vi "AprilTag Target Package.vi"() -> ()   [LabVIEW 2023]
uses:
  Camera Info.ctl
  AprialTag Main Cluster.ctl
  AprialTag States.ctl
  <vilib>/vision/Image Controls.llb/IMAQ Image.ctl
  Camera Set Up/Event Setup Types.ctl
  <vilib>/Utility/config.llb/Read Key (String).vi
  <vilib>/Utility/config.llb/Write Key (String).vi
  <vilib>/Utility/config.llb/NI_LVConfig.lvlib
panel:
  in  "Main":enum32{"Page 1", "Page 2"}(tab)
  out "Tag ID":dbl[](array[numeric]) caption="Tag Number"
  out "Image":T1(plugin-control)
  in  "Camera Name":string="cam0"
  in  "Settings":bool
  in  "Save":bool
  in  "Tools":bool
  out "Fps":dbl format="%#.0f"
  out "Distance":dbl[](array[numeric]) format="%.1f"
  out "Angle":dbl[](array[numeric]) format="%.1f"
  in  "Home":bool
  in  "FOV":dbl=68.5
  in  "Robot Calibration Cluster":T2={"Camera Height on robot (in)"=9.5, "Camera Angle on the robot (deg)"=2.5, "Camera FOV Top to Bottom View Angle (deg)"=26.5, "Target size (in)"=6.5, "Distance to front of bumper (in)"=9.75} {"Distance to front of bumper (in)" format="%#_13g"; "Target size (in)" format="%#_13g"; "Camera FOV Top to Bottom View Angle (deg)" format="%#_13g"; "Camera Angle on the robot (deg)" format="%#_13g"; "Camera Height on robot (in)" format="%#_13g"}
  # "Edit the camera name to the camera that you are going to use for this target package"
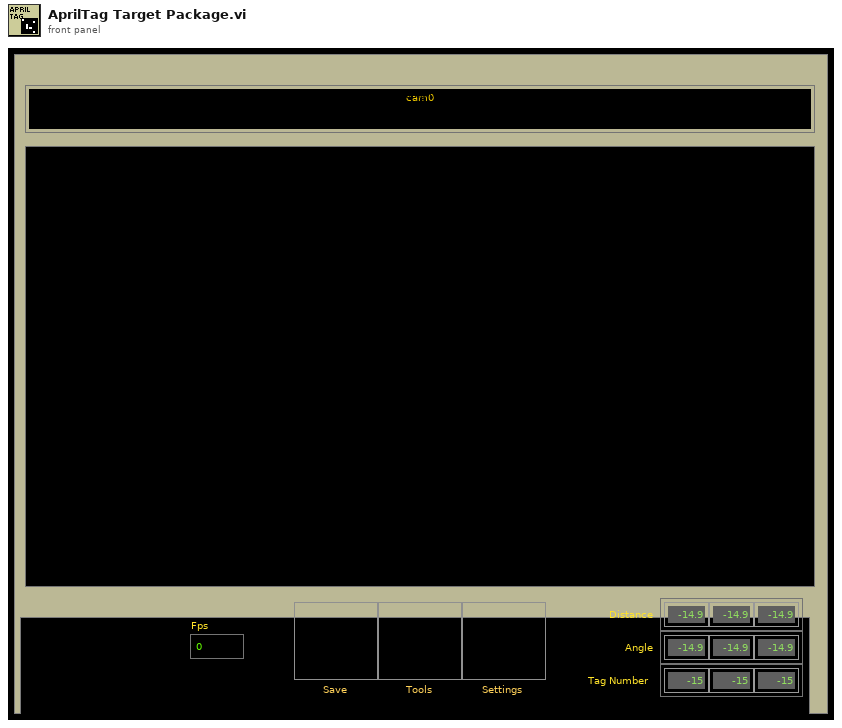
[diagram p1: front panel]
types:
  T1 = typedef "IMAQ Image.ctl" = refnum<image>
  T2 = typedef "Camera Info.ctl" = cluster{"Camera Height on robot (in)":dbl, "Camera Angle on the robot (deg)":dbl, "Camera FOV Top to Bottom View Angle (deg)":dbl, "Target size (in)":dbl, "Distance to front of bumper (in)":dbl}
  T3 = typedef "AprialTag States.ctl" = enum16{"Message Dispatcher", "INI", "Open", "Save", "Exit"}
  T4 = typedef "AprialTag Main Cluster.ctl" = cluster{"AprilTage FIFO":T3[], "Camera Name":string, "AprilTag path":path, "Control Ref's":refnum<vi>[], "Greyscale Mask Image":T1, "Main Image":T1}
  T5 = typedef "Event Setup Types.ctl" = enum16{"Default", "Camera Loop Started", "Save Data", "Open Front Panel", "Exit"}
  T6 = typedef "Image Type" = u32
  T7 = cluster{"tag ID":i32, "Center":cluster{"X":dbl, "Y":dbl}, "homography matrix":dbl[], "decision margin":dbl, "Hamming Dist":i32, "corner points":cluster{"X":dbl, "Y":dbl}[], "Tag Family":string}[]
  T8 = typedef "AprilTag Target Fields.ctl" = cluster{"diameter points":cluster{"first point":cluster{"x":dbl, "y":dbl}, "projected point":cluster{"x":dbl, "y":dbl}}, "normalized center":cluster{"x":dbl, "y":dbl}, "Overall Score":dbl, "Distance (ft)":dbl, "Target corner points":cluster{"X":dbl, "Y":dbl}[], "Target Center":cluster{"X":dbl, "Y":dbl}}
  T9 = typedef "NI_LVConfig.lvlib/Config Data RefNum.ctl" = refnum<k1>
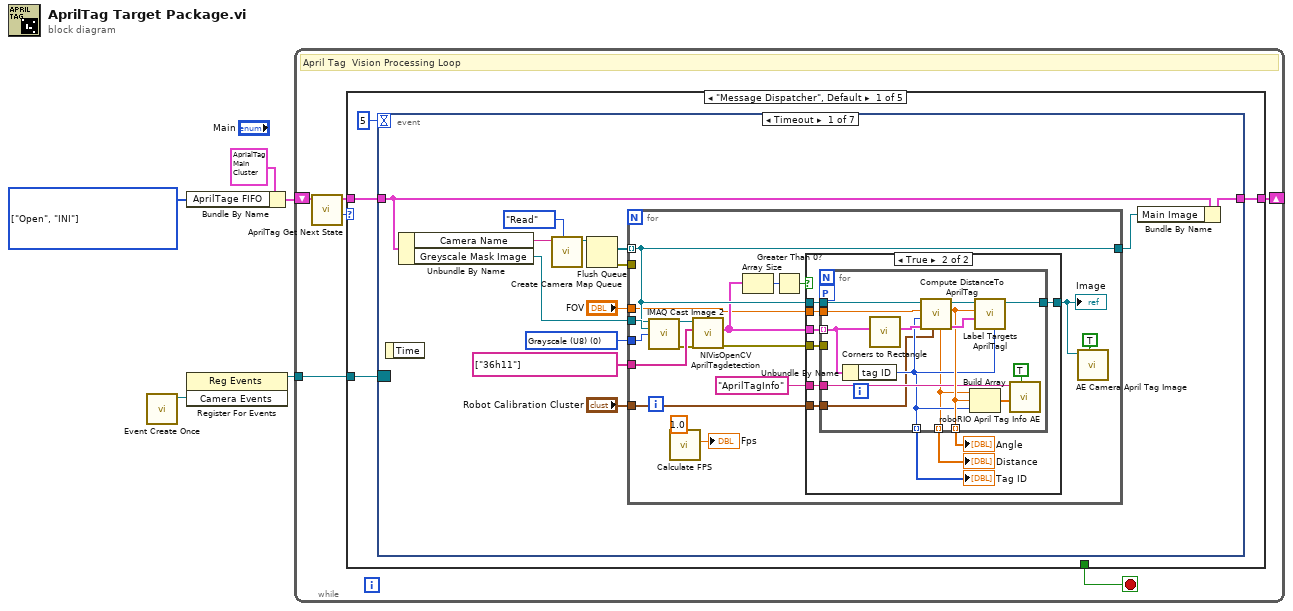
[diagram p0: block diagram]
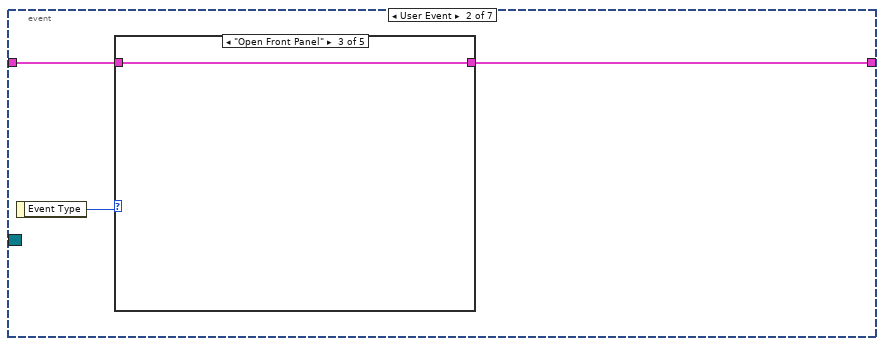
[diagram p3: hidden frame]
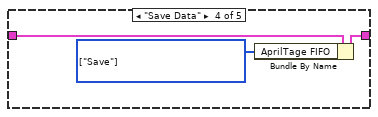
[diagram p6: hidden frame]
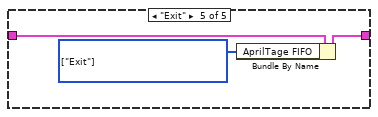
[diagram p7: hidden frame]
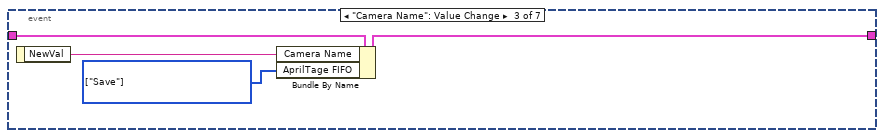
[diagram p8: hidden frame]
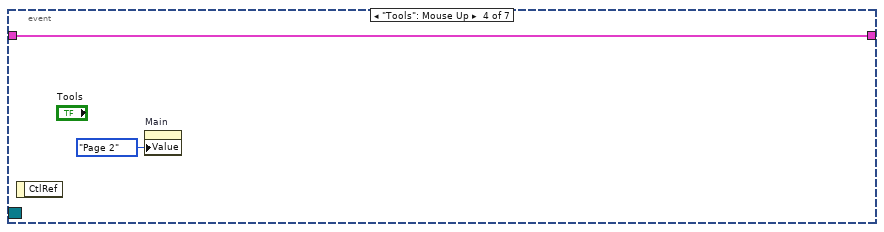
[diagram p9: hidden frame]
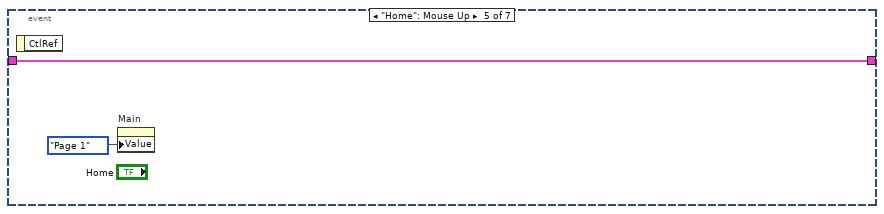
[diagram p10: hidden frame]
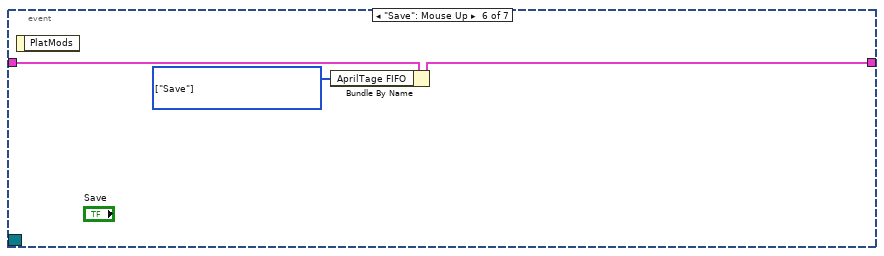
[diagram p11: hidden frame]
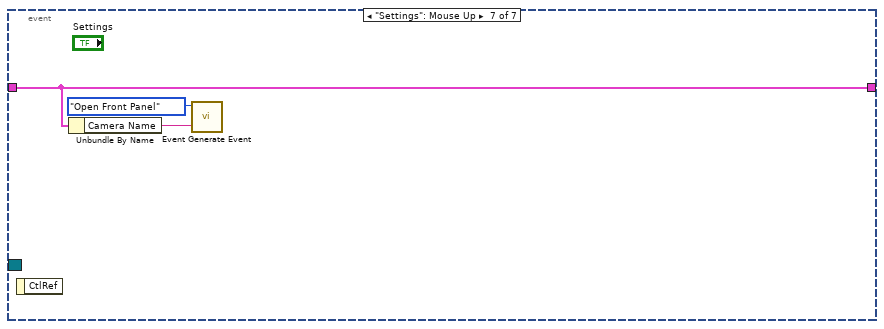
[diagram p12: hidden frame]
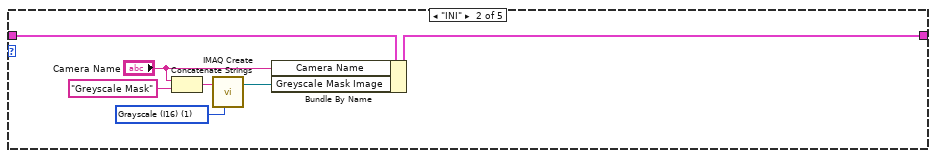
[diagram p13: hidden frame]
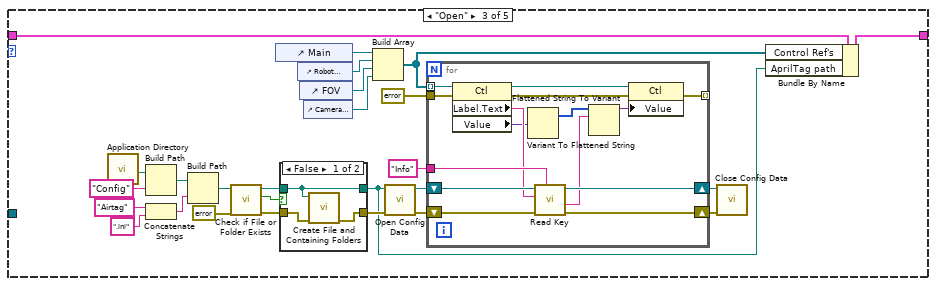
[diagram p14: hidden frame]
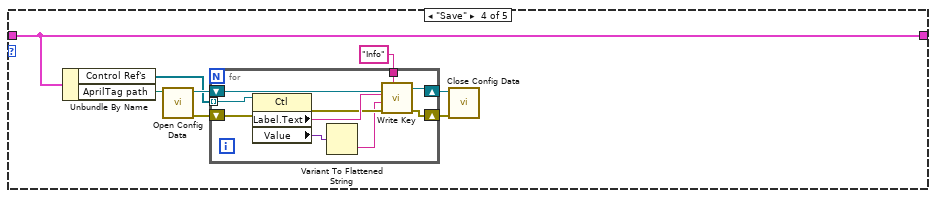
[diagram p16: hidden frame]
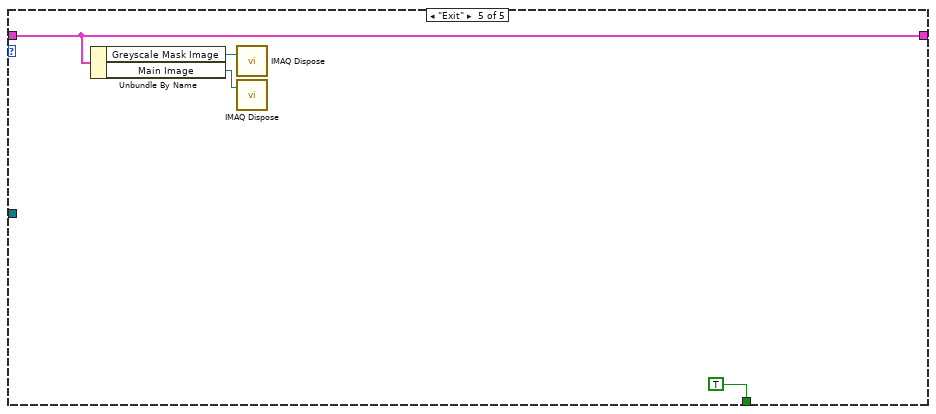
[diagram p17: hidden frame]
diagram:
  w1 = T3[] [enum."Open", enum."INI"] items=["Message Dispatcher", "INI", "Open", "Save", "Exit"] ("AprilTage FIFO")
  n1 = call "Event Create Once.vi"() -> ("Camera Events"=w5:refnum<user-event>)  [unwired: 10 in, 1 out]
  n2 = Bundle By Name(cluster=T4 {"AprilTage FIFO"=[], "Camera Name"="", "AprilTag path"=path "", "Control Ref's"=[], "Greyscale Mask Image"=refnum, "Main Image"=refnum} ("AprilTag Main Cluster out"), "AprilTage FIFO"=w1) -> (w2:T4)
  n3 = register-events(w5) -> (reference out=w4:refnum<event-registration>)  [unwired: 2 in, 1 out]
  n4 = while {
    tunnel: w4 -> [w11]
    shift-right: [w6] -> _
    shift-left: w2 -> [w9]
    stop <- w10 stop-if-true
    # "April Tag  Vision Processing Loop"
    n5 = call "AprilTag Get Next State.vi"("AprilTag Main Cluster in"=w9) -> ("Next State"=w7:T3, "AprilTag Main Cluster out"=w8:T4)  [unwired: 9 in]
    n6 = case shown="\"Message Dispatcher\", Default" w7 {
      tunnel: w11 -> [w15 _ _ _ _]
      tunnel: [_ _ _ _ TRUE] -> w10
      tunnel: w8 -> [w13 w103 w115 w153 w170]
      tunnel: [w12 w102 w113 w153 w170] -> w6
      frame "Message Dispatcher", Default {
        n7 = event shown="[0] Timeout" {
          selector: w15 -> [_ _ _ _ _ _ _]
          dyn-events: _ -> [_ _ _ _ _ _ _]
          timeout: 5 -> [_ _ _ _ _ _ _]
          tunnel: w13 -> [w21 w73 w86 w87 w89 w93 w95]
          tunnel: [w18 w72 w85 w87 w89 w92 w95] -> w12
          event Timeout {
            w26 = T6 0 items=["Grayscale (U8)", "Grayscale (I16)", "Grayscale (SGL)", "Complex (CSG)", "RGB (U32)", "HSL (U32)", "RGB (U64)", "Grayscale (U16)"] ("Image Type")
            n8 = event-data() -> ()  [unwired: 1 in, 1 out]
            n9 = Unbundle By Name(w21) -> ("Camera Name"=w20:string, "Greyscale Mask Image"=w19:T1)
            n10 = call "Create Camera Map Queue.vi"("Action"=enum16{"Read", "Write"}."Read", "Camera"=w20) -> ("value"=w27:refnum<queue>)  [unwired: 8 in, 1 out]
            n11 = Flush Queue(queue=w27) -> (remaining elements=w25:T1[], error out=w16:errorcluster)  [unwired: 1 in, 1 out]
            n12 = for {
              tunnel: w19 -> [w45]
              tunnel: w25 -> [w43] mode=indexing
              tunnel: w26 -> [w44]
              tunnel: [w43] -> w17
              tunnel: string[] ["36h11"] ("Tag Familys") -> [w42]
              tunnel: "FOV" -> [w33]
              tunnel: "Robot Calibration Cluster" -> [w32]
              tunnel: w16 -> [_]
              n13 = call "IMAQ Cast Image 2"("Image Src"=w43, "Image Dst"=w45, "Image Type"=w44) -> ("Image Dst Out"=w41:T1, "error out"=w36:errorcluster)  [unwired: 11 in]
              n14 = call "Calculate FPS.vi"("Frames Processed"=1.0) -> ("Fps"=→"Fps":dbl)  [unwired: 10 in]
              n15 = call "NIVisOpenCV AprilTagdetection.vi"("error in (no error)"=w36, "Tag Familys"=w42, "Image Src"=w41) -> ("error out"=w35:errorcluster, "Detected Tags"=w39:T7)  [unwired: 5 in, 2 out]
              n16 = Array Size(array=w39) -> (size(s)=w38:i32)
              n17 = Greater Than 0?(x=w38) -> (x > 0?=w37:bool)
              n18 = case shown="True" w37 {
                tunnel: w43 -> [w46 w56]
                tunnel: w39 -> [_ w55]
                tunnel: [w46 w54] -> w40
                tunnel: w35 -> [_ w53]
                tunnel: "AprilTagInfo" ("Name") -> [_ w49]
                tunnel: w33 -> [_ w48]
                tunnel: w32 -> [_ w47]
                frame False {
                }
                frame True {
                  n19 = for {
                    tunnel: w55 -> [w68] mode=indexing
                    tunnel: w56 -> [w69]
                    tunnel: [w70] -> w54
                    tunnel: w53 -> [_]
                    tunnel: [w59] -> w52 mode=indexing
                    tunnel: [w57] -> w51 mode=indexing
                    tunnel: [w63] -> w50 mode=indexing
                    tunnel: w49 -> [w61]
                    tunnel: w48 -> [w60]
                    tunnel: w47 -> [w58]
                    workers-P: _ -> [_]
                    n20 = Unbundle By Name(w68) -> ("tag ID"=w59:i32)
                    n21 = call "Corners to Rectangle.vi"("tag info"=w68) -> ("output cluster"=w67:T8)  [unwired: 10 in]
                    n22 = call "Compute DistanceTo AprilTag.vi"("Robot Calibration Cluster"=w58, "results"=w67, "AprilTag Number"=w59, "FOV Left to Right (deg)"=w60, "Image Src"=w69) -> ("results out"=w66:T8, "Offset Angle"=w63:dbl, "Image Dst Out"=w65:T1, "Distance from target (in)"=w57:dbl)  [unwired: 3 in]
                    n23 = Build Array(w57, w63, w59) -> (w62:dbl[])
                    n24 = call "Label Targets AprilTagl.vi"("AprilTag Number"=w59, "results"=w66, "Angle"=w63, "Image in"=w65) -> ("Image out"=w70:T1)  [unwired: 7 in]
                    n25 = call "roboRIO April Tag Info AE.vi"("Update"=TRUE, "Info in"=w62, "name"=w61) -> ()  [unwired: 8 in, 1 out]
                  }
                  "Distance" <- w51
                  "Angle" <- w50
                  "Tag ID" <- w52
                }
              }
              "Image" <- w40
              n26 = call "AE Camera April Tag Image.vi"("Update"=TRUE, "Ball Image in"=w40) -> ()  [unwired: 9 in, 1 out]
            }
            n27 = Bundle By Name(cluster=w21, "Main Image"=w17) -> (w18:T4)
          }
          event User Event {
            n28 = event-data() -> ("Event Type"=w71:T5)  [unwired: 1 in]
            n29 = case shown="\"Open Front Panel\"" w71 {
              tunnel: w73 -> [w74 w75 w76 w79 w82]
              tunnel: [w74 w75 w76 w78 w81] -> w72
              frame "Default" {
              }
              frame "Camera Loop Started" {
              }
              frame "Open Front Panel" {
              }
              frame "Save Data" {
                w77 = T3[] [enum."Save"] items=["Message Dispatcher", "INI", "Open", "Save", "Exit"] ("AprilTage FIFO")
                n30 = Bundle By Name(cluster=w79, "AprilTage FIFO"=w77) -> (w78:T4)
              }
              frame "Exit" {
                w80 = T3[] [enum."Exit"] items=["Message Dispatcher", "INI", "Open", "Save", "Exit"] ("AprilTage FIFO")
                n31 = Bundle By Name(cluster=w82, "AprilTage FIFO"=w80) -> (w81:T4)
              }
            }
          }
          event "Camera Name": Value Change {
            w84 = T3[] [enum."Save"] items=["Message Dispatcher", "INI", "Open", "Save", "Exit"] ("AprilTage FIFO")
            n32 = event-data() -> ("NewVal"=w83:string)  [unwired: 1 in]
            n33 = Bundle By Name(cluster=w86, "Camera Name"=w83, "AprilTage FIFO"=w84) -> (w85:T4)
          }
          event "Tools": Mouse Up {
            n34 = event-data() -> ()  [unwired: 1 in, 1 out]
            n35 = property on="Main" class="TabCtl (strict)"("Value"=enum32{"Page 1", "Page 2"}."Page 2" ("Main")) -> ()  [unwired: 2 in, 2 out]
          }
          event "Home": Mouse Up {
            n36 = event-data() -> ()  [unwired: 1 in, 1 out]
            n37 = property on="Main" class="TabCtl (strict)"("Value"=enum32{"Page 1", "Page 2"}."Page 1" ("Main")) -> ()  [unwired: 2 in, 2 out]
          }
          event "Save": Mouse Up {
            w91 = T3[] [enum."Save"] items=["Message Dispatcher", "INI", "Open", "Save", "Exit"] ("AprilTage FIFO")
            n38 = event-data() -> ()  [unwired: 1 in, 1 out]
            n39 = Bundle By Name(cluster=w93, "AprilTage FIFO"=w91) -> (w92:T4)
          }
          event "Settings": Mouse Up {
            n40 = event-data() -> ()  [unwired: 1 in, 1 out]
            n41 = Unbundle By Name(w95) -> ("Camera Name"=w94:string)
            n42 = call "Event Generate Event.vi"("Camera Name"=w94, "Event Type"=Event_Setup_Types."Open Front Panel") -> ()  [unwired: 10 in]
          }
        }
      }
      frame "INI" {
        w99 = T6 1 items=["Grayscale (U8)", "Grayscale (I16)", "Grayscale (SGL)", "Complex (CSG)", "RGB (U32)", "HSL (U32)", "RGB (U64)", "Grayscale (U16)"] ("Image Type")
        n43 = Concatenate Strings("Camera Name", "Greyscale Mask" ("string")) -> (w100:string)
        n44 = call "IMAQ Create"("Image Name"=w100, "Image Type"=w99) -> ("New Image"=w98:T1)  [unwired: 2 in, 2 out]
        n45 = Bundle By Name(cluster=w103, "Camera Name"="Camera Name", "Greyscale Mask Image"=w98) -> (w102:T4)
      }
      frame "Open" {
        n46 = call <vilib>:"Application Directory.vi"() -> ("Application Directory"=w118:path)
        n47 = Build Path(base path=w118, name or relative path="Config") -> (appended path=w116:path)
        n48 = Concatenate Strings("Airtag" ("string"), ".ini" ("name or relative path")) -> (w129:string)
        n49 = Build Path(base path=w116, name or relative path=w129) -> (appended path=w109:path)
        n50 = call <vilib>:"Check if File or Folder Exists.vi"("error in (no error)"=errorcluster {"status"=FALSE, "code"=0, "source"=""}, "path"=w109) -> ("error out"=w105:errorcluster, "file or folder exists?"=w107:bool, "dup path"=w108:path)  [unwired: 7 in]
        n51 = control-ref of="Main"() -> (w124:refnum<vi>)
        n52 = case shown="False" w107 {
          tunnel: [w132 w133] -> w119
          tunnel: w108 -> [w131 w134]
          tunnel: [w131 w134] -> w106
          tunnel: w105 -> [w130 w133]
          frame False {
            n53 = call <vilib>:"Create File and Containing Folders.vi"("error in (no error)"=w130, "file path"=w131) -> ("error out"=w132:errorcluster)  [unwired: 8 in, 1 out]
          }
          frame True {
          }
        }
        n54 = control-ref of="Robot Calibration Cluster"() -> (w123:refnum<vi>)
        n55 = control-ref of="FOV"() -> (w122:refnum<vi>)
        n56 = control-ref of="Camera Name"() -> (w114:refnum<vi>)
        n57 = Build Array(w124, w123, w122, w114) -> (w112:refnum<vi>[])
        n58 = call <vilib>:"Open Config Data.vi"("error in (no error)"=w119, "configuration file path"=w106) -> ("error out"=w125:errorcluster, "refnum"=w128:T9)  [unwired: 7 in, 1 out]
        n59 = for {
          tunnel: "Info" ("Camera Name") -> [w146]
          tunnel: w112 -> [w144] mode=indexing
          shift-right: [w148] -> w127
          shift-left: w128 -> [w149]
          shift-right: [w147] -> w126
          shift-left: w125 -> [w145]
          tunnel: [w139] -> _ mode=indexing
          tunnel: errorcluster {"status"=FALSE, "code"=0, "source"=""} ("error out") -> [w138]
          n60 = property class="Ctl"(reference=w144, error in=w138) -> (reference out=w142:refnum<vi>, error out=w140:errorcluster, "Label.Text"=w143:string, "Value"=w136:variant)
          n61 = Variant To Flattened String(Variant=w136) -> (1:w135:i16[])  [unwired: 1 out]
          n62 = call-poly <vilib>:"Read Key.vi"("section"=w146, "error in (no error)"=w145, "key"=w143, "refnum"=w149) -> ("error out"=w147:errorcluster, "value"=w141:string, "refnum out"=w148:T9)  [unwired: 4 in, 1 out]
          n63 = Flattened String To Variant(6:w141, 7:w135) -> (3:w137:variant)  [unwired: 1 in, 1 out]
          n64 = property class="Ctl"(reference=w142, error in=w140, "Value"=w137) -> (error out=w139:errorcluster)  [unwired: 1 out]
        }
        n65 = call <vilib>:"Close Config Data.vi"("error in (no error)"=w126, "refnum"=w127) -> ()  [unwired: 8 in, 2 out]
        n66 = Bundle By Name(cluster=w115, "Control Ref's"=w112, "AprilTag path"=w106) -> (w113:T4)
      }
      frame "Save" {
        n67 = Unbundle By Name(w153) -> ("Control Ref's"=w151:refnum<vi>[], "AprilTag path"=w152:path)
        n68 = call <vilib>:"Open Config Data.vi"("configuration file path"=w152) -> ("error out"=w154:errorcluster, "refnum"=w157:T9)  [unwired: 8 in, 1 out]
        n69 = for {
          tunnel: "Info" ("Camera Name") -> [w163]
          shift-right: [w166] -> w156
          shift-left: w157 -> [w167]
          shift-right: [w165] -> w155
          shift-left: w154 -> [w164]
          tunnel: w151 -> [w158] mode=indexing
          n70 = property class="Ctl"(reference=w158, error in=w164) -> (error out=w160:errorcluster, "Label.Text"=w162:string, "Value"=w161:variant)  [unwired: 1 out]
          n71 = Variant To Flattened String(Variant=w161) -> (data string=w159:string)  [unwired: 1 out]
          n72 = call-poly <vilib>:"Write Key.vi"("section"=w163, "error in (no error)"=w160, "value"=w159, "key"=w162, "refnum"=w167) -> ("error out"=w165:errorcluster, "refnum out"=w166:T9)  [unwired: 4 in, 1 out]
        }
        n73 = call <vilib>:"Close Config Data.vi"("error in (no error)"=w155, "refnum"=w156) -> ()  [unwired: 8 in, 2 out]
      }
      frame "Exit" {
        n74 = Unbundle By Name(w170) -> ("Greyscale Mask Image"=w169:T1, "Main Image"=w168:T1)
        n75 = call "IMAQ Dispose"("Image"=w169) -> ()  [unwired: 5 in, 1 out]
        n76 = call "IMAQ Dispose"("Image"=w168) -> ()  [unwired: 5 in, 1 out]
      }
    }
  }
